vi "Grid_Adam7.vi"(7 "reset":bool, 10 "py 2":i64=24, 11 "px 2":i64=24) -> (2 "index of element":i32=292, 3 "initinalized":bool)   [LabVIEW 2021]
panel:
  out "pattern array":i32[](array[numeric])
  in  "adam7 2":i32[][](array[numeric])=[[1, 6, 4, 6, 2, 6, 4, 6], [7, 7, 7, 7, 7, 7, 7, 7], [5, 6, 5, 6, 5, 6, 5, 6], [7, 7, 7, 7, 7, 7, 7, 7], [3, 6, 4, 6, 3, 6, 4, 6], [7, 7, 7, 7, 7, 7, 7, 7], [5, 6, 5, 6, 5, 6, 5, 6], [7, 7, 7, 7, 7, 7, 7, 7]]
  in  "index":i64=293
  in  "number7":i64=3
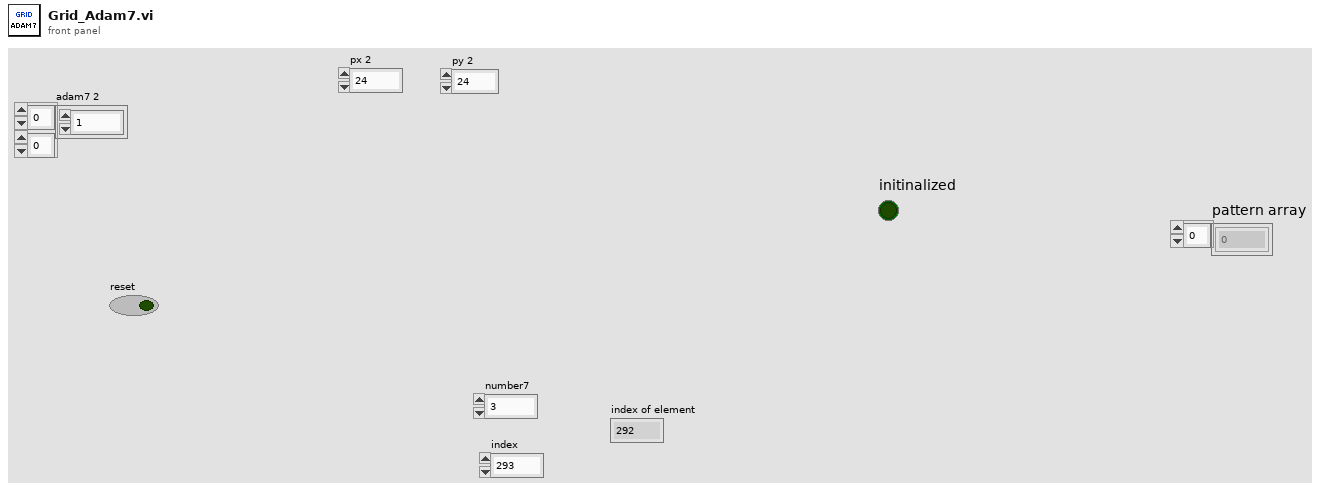
[diagram p1: front panel]
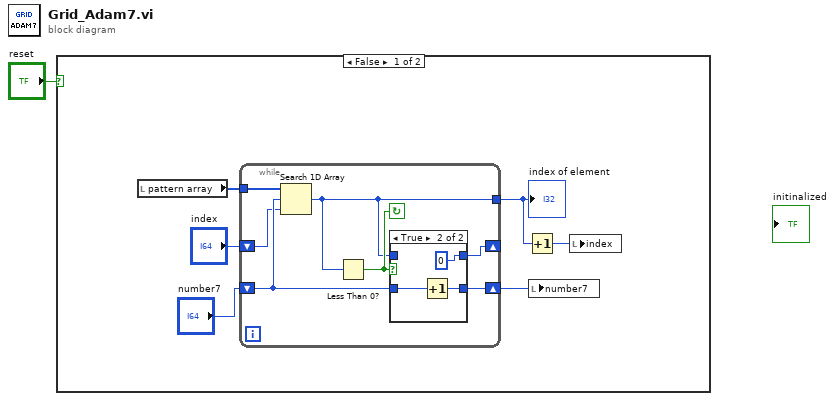
[diagram p0: block diagram]
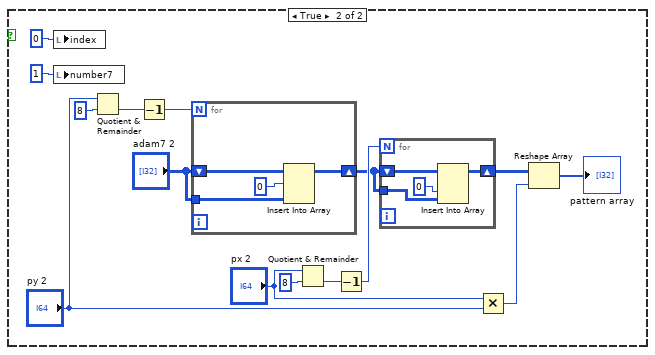
[diagram p3: hidden frame]
diagram:
  n1 = case shown="False" "reset" {
    frame False {
      n2 = local read "pattern array"() -> (w2:i32[])
      n3 = while {
        tunnel: w2 -> [w14]
        tunnel: [w8] -> w3
        shift-right: [w12] -> w5
        shift-left: "number7" -> [w11]
        shift-right: [w10] -> _
        shift-left: "index" -> [w9]
        stop <- w13 continue-if-true
        n4 = Search 1D Array(1D array=w14, element=w11, start index (0)=w9) -> (index of element=w8:i32)
        n5 = Less Than 0?(x=w8) -> (x < 0?=w13:bool)
        n6 = case shown="True" w13 {
          tunnel: w11 -> [w16 w19]
          tunnel: [w16 w18] -> w12
          tunnel: [w15 i64 0 ("start index (0)")] -> w10
          tunnel: w8 -> [w15 _]
          frame False {
          }
          frame True {
            n7 = Increment(x=w19) -> (x+1=w18:i64)
          }
        }
      }
      "index of element" <- w3
      n8 = Increment(x=w3) -> (x+1=w4:i32)
      n9 = local write "number7"(w5) -> ()
      n10 = local write "index"(w4) -> ()
    }
    frame True {
      n11 = local write "index"(i64 0 ("index")) -> ()
      n12 = local write "number7"(i64 1 ("number7")) -> ()
      n13 = Quotient & Remainder(x="py 2", y=i64 8) -> (floor(x/y)=w26:i64)  [unwired: 1 out]
      n14 = Decrement(x=w26) -> (x-1=w29:i64)
      n15 = for {
        N: w29 -> [_]
        shift-right: [w40] -> w22
        shift-left: "adam7 2" -> [w41]
        tunnel: "adam7 2" -> [w39]
        n16 = Insert Into Array(array=w41, index (row)=0, new element=w39) -> (w40:i32[][])  [unwired: 1 in]
      }
      n17 = Quotient & Remainder(x="px 2", y=i64 8) -> (floor(x/y)=w27:i64)  [unwired: 1 out]
      n18 = Decrement(x=w27) -> (x-1=w28:i64)
      n19 = for {
        N: w28 -> [_]
        shift-right: [w37] -> w24
        shift-left: w22 -> [w38]
        tunnel: w22 -> [w35]
        n20 = Insert Into Array(array=w38, index (col)=0 ("index (row)"), new element=w35) -> (w37:i32[][])  [unwired: 1 in]
      }
      n21 = Multiply(x="px 2", y="py 2") -> (x*y=w21:i64)
      n22 = Reshape Array(w24, w21) -> (→"pattern array":i32[])
    }
  }
